vi "Get 摄像头电源.vi"(11 "DAM0200-Relay in":refnum<class "DAM0200-Relay.lvclass">) -> (2 "摄像头电源":refnum<vi>, 3 "DAM0200-Relay out":refnum<class "DAM0200-Relay.lvclass">)   [LabVIEW 2016, in "DAM0200-Relay.lvlib" / "DAM0200-Relay.lvclass"]
uses:
  DAM0200-Relay.lvclass
  DAM0200-Relay.lvclass/DAM0200-Relay.ctl
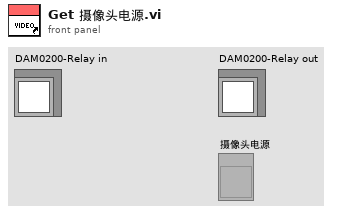
[diagram p1: front panel]
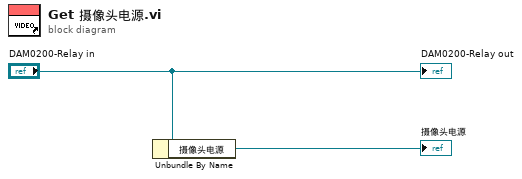
[diagram p0: block diagram]
diagram:
  n1 = Unbundle By Name("DAM0200-Relay in") -> ("摄像头电源"=→"摄像头电源":refnum<vi>)
  "DAM0200-Relay out" <- "DAM0200-Relay in"
